vi "Sample in Container.vi"(8 "error in (no error)":errorcluster, 10 "Container":T1, 11 "cRIO-CO2 in":refnum<class "cRIO-CO2.lvclass">) -> (0 "error out":errorcluster, 2 "Sample":refnum<class "Sample.lvclass">, 3 "cRIO-CO2 out":refnum<class "cRIO-CO2.lvclass">)   [LabVIEW 2015, in "cRIO-Carbondioxide.lvlib" / "cRIO-CO2.lvlib" / "cRIO-CO2.lvclass"]
uses:
  cRIO-CO2.lvclass
  Controls/Sample Transfer Container Enumerator.ctl
  subs/Sample/Sample.lvclass
  cRIO-CO2.lvclass/cRIO-CO2.ctl
  Sample Line/Sample Line.lvclass
  Controls/Sample Line State Enumerator.ctl
  CO2 Actor Messages/Ping Msg/Ping Msg.lvclass/Ping Msg.ctl
  <vilib>/ActorFramework/Message Enqueuer/Message Enqueuer.lvclass/Message Enqueuer.ctl
  Storage Line/Storage Line.lvclass
  Storage Line/Storage Line.lvclass/Storage Line.ctl
  Syringe Line/Syringe Line.lvclass
  <vilib>/ActorFramework/Message Enqueuer/Enqueue.vi
  <vilib>/ActorFramework/Message Priority Queue/Priority Enqueue.vi
  <vilib>/ActorFramework/Message Enqueuer/Message Enqueuer.lvclass
  CO2 Actor Messages/Ping Msg/Ping Msg.lvclass
  <vilib>/ActorFramework/Actor/Actor.lvclass
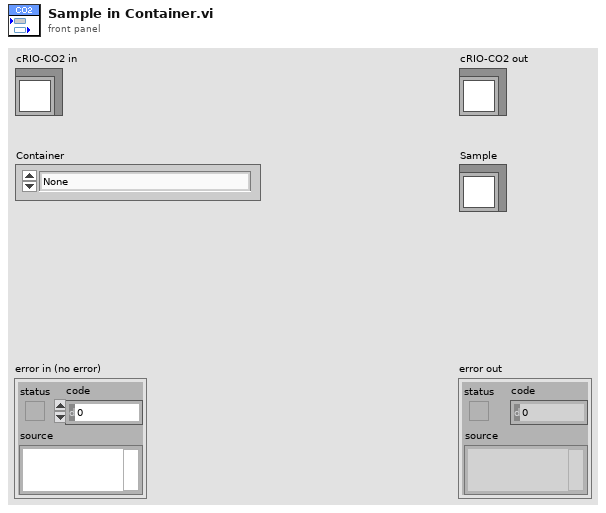
[diagram p1: front panel]
types:
  T1 = typedef "Sample Transfer Container Enumerator.ctl" = enum16{"None", "Sample 1", "Sample 2", "Sample 3", "Sample 4", "Sample 5", "Storage 01", "Storage 02", "Storage 03", "Storage 04", "Storage 05", "Storage 06", "Storage 07", "Storage 08", "Storage 09", "Storage 10", "Storage 11", "Storage 12", "Syringe", "Undefined"}
  T2 = typedef "Sample Line State Enumerator.ctl" = enum16{"All lines closed", "Sample line 1.", "Sample line 2.", "Sample line 3.", "Sample line 4.", "Sample line 5.", "Out of range"}
  T3 = typedef "Dedicated Enqueuers.ctl" = cluster{"Freezers":cluster{"Syringe":refnum<class "Message Enqueuer.lvclass">, "Tank 1":refnum<class "Message Enqueuer.lvclass">, "Tank 2":refnum<class "Message Enqueuer.lvclass">, "Tank 3":refnum<class "Message Enqueuer.lvclass">, "Tank 4":refnum<class "Message Enqueuer.lvclass">}, "Heaters":cluster{"Syringe":refnum<class "Message Enqueuer.lvclass">, "Piston":refnum<class "Message Enqueuer.lvclass">}, "Blowers":cluster{"Tank 1":refnum<class "Message Enqueuer.lvclass">, "Tank 2":refnum<class "Message Enqueuer.lvclass">, "Tank 3":refnum<class "Message Enqueuer.lvclass">, "Tank 4":refnum<class "Message Enqueuer.lvclass">, "Syringe":refnum<class "Message Enqueuer.lvclass">}, "Sample Line":refnum<class "Message Enqueuer.lvclass">, "Storage Line":refnum<class "Message Enqueuer.lvclass">, "Transfer Line":refnum<class "Message Enqueuer.lvclass">, "Syringe Stepper":refnum<class "Message Enqueuer.lvclass">, "Syringe Line":refnum<class "Message Enqueuer.lvclass">, "Capillary Line":refnum<class "Message Enqueuer.lvclass">, "Preparation Line":refnum<class "Message Enqueuer.lvclass">, "Turbo":refnum<class "Message Enqueuer.lvclass">, "Vacuum":refnum<class "Message Enqueuer.lvclass">, "He Line":refnum<class "Message Enqueuer.lvclass">, "Cylinder":refnum<class "Message Enqueuer.lvclass">}
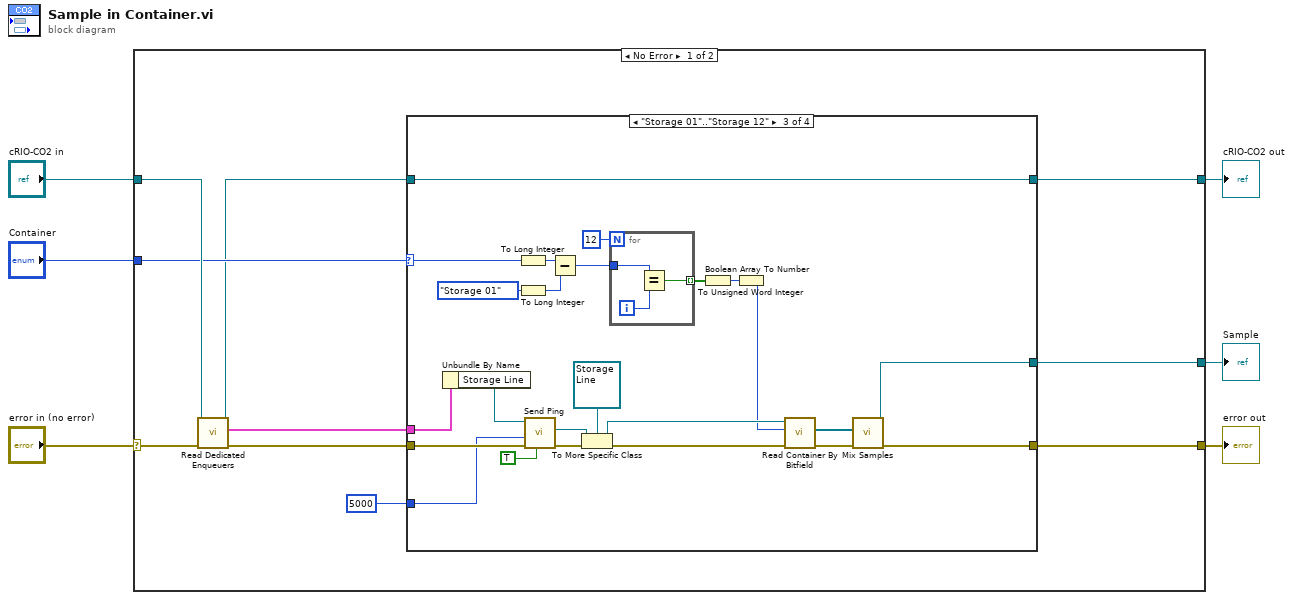
[diagram p0: block diagram]
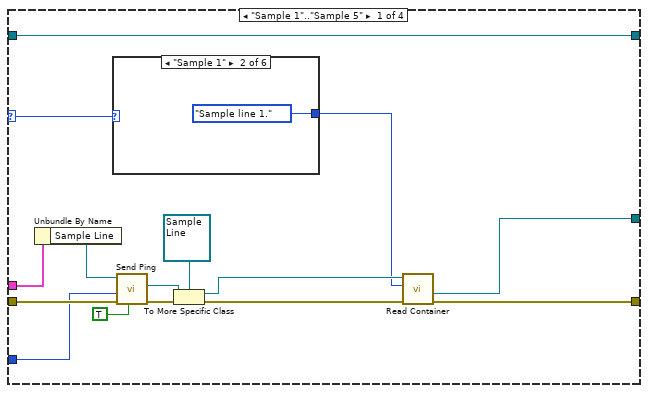
[diagram p2: hidden frame]
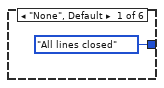
[diagram p3: hidden frame]
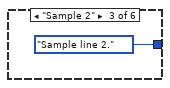
[diagram p4: hidden frame]
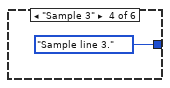
[diagram p5: hidden frame]
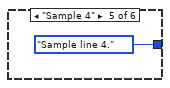
[diagram p6: hidden frame]
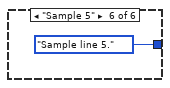
[diagram p7: hidden frame]
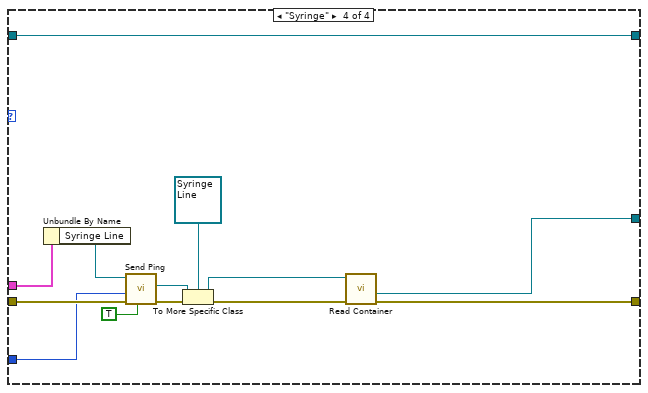
[diagram p9: hidden frame]
diagram:
  n1 = case shown="No Error" "error in (no error)" {
    selector: "error in (no error)" -> [w16 w81]
    tunnel: [w8 w81] -> w5
    tunnel: [w12 w80] -> w3
    tunnel: "cRIO-CO2 in" -> [w15 w80]
    tunnel: "Container" -> [w13 _]
    tunnel: [w7 _] -> w1
    frame No Error {
      n2 = call "Read Dedicated Enqueuers.vi"("error in (no error)"=w16, "cRIO-CO2 in"=w15) -> ("error out"=w14:errorcluster, "Dedicated Enqueuers"=w10:T3, "cRIO-CO2 out"=w11:refnum<class "cRIO-CO2.lvclass">)  [unwired: 6 in, 1 out]
      n3 = case shown="\"Storage 01\"..\"Storage 12\"" w13 {
        selector: w13 -> [w18 _ w49 _]
        tunnel: w14 -> [w30 w39 w59 w76]
        tunnel: [w24 w39 w54 w71] -> w8
        tunnel: [w23 _ w40 w72] -> w7
        tunnel: w10 -> [w31 _ w58 w75]
        tunnel: 5000 ("timeout in ms (1000)") -> [w22 _ w53 w70]
        tunnel: [w21 w38 w52 w69] -> w12
        tunnel: w11 -> [w21 w38 w52 w69]
        frame "Sample 1".."Sample 5" {
          n4 = Unbundle By Name(w31) -> ("Sample Line"=w29:refnum<class "Message Enqueuer.lvclass">)
          n5 = case shown="\"Sample 1\"" w18 {
            tunnel: [Sample_Line_State_Enumerator."All lines closed" ("Sample Line (All Closed)") Sample_Line_State_Enumerator."Sample line 1." ("Sample Line (All Closed)") Sample_Line_State_Enumerator."Sample line 2." ("Sample Line (All Closed)") Sample_Line_State_Enumerator."Sample line 3." ("Sample Line (All Closed)") Sample_Line_State_Enumerator."Sample line 4." ("Sample Line (All Closed)") Sample_Line_State_Enumerator."Sample line 5." ("Sample Line (All Closed)")] -> w17
            frame "None", Default {
            }
            frame "Sample 1" {
            }
            frame "Sample 2" {
            }
            frame "Sample 3" {
            }
            frame "Sample 4" {
            }
            frame "Sample 5" {
            }
          }
          n6 = call "Send Ping.vi"("Return Self (F)"=TRUE, "error in (no error)"=w30, "timeout in ms (1000)"=w22, "Message Enqueuer"=w29) -> ("error out"=w27:errorcluster, "Actor out"=w25:refnum<class "Actor.lvclass">)  [unwired: 4 in, 2 out]
          n7 = To More Specific Class(target class=refnum<class "Sample Line.lvclass"> refnum ("Sample Line in"), reference=w25, error in=w27) -> (specific class reference=w19:refnum<class "Sample Line.lvclass">, error out=w20:errorcluster)
          n8 = call "Read Container.vi"("error in (no error)"=w20, "Sample Line (All Closed)"=w17, "Sample Line in"=w19) -> ("error out"=w24:errorcluster, "Sample"=w23:refnum<class "Sample.lvclass">)  [unwired: 5 in, 2 out]
        }
        frame "None", "Undefined" {
        }
        frame "Storage 01".."Storage 12" {
          n9 = Unbundle By Name(w58) -> ("Storage Line"=w63:refnum<class "Message Enqueuer.lvclass">)
          n10 = To Long Integer(number=w49) -> (32bit integer=w48:i32)
          n11 = To Long Integer(number=Sample_Transfer_Container_Enumerator."Storage 01" ("Container")) -> (32bit integer=w46:i32)
          n12 = call "Send Ping.vi"("Return Self (F)"=TRUE, "error in (no error)"=w59, "timeout in ms (1000)"=w53, "Message Enqueuer"=w63) -> ("error out"=w61:errorcluster, "Actor out"=w60:refnum<class "Actor.lvclass">)  [unwired: 4 in, 2 out]
          n13 = Subtract(x=w48, y=w46) -> (x-y=w45:i32)
          n14 = To More Specific Class(target class=refnum<class "Storage Line.lvclass"> refnum ("Storage Line in"), reference=w60, error in=w61) -> (specific class reference=w51:refnum<class "Storage Line.lvclass">, error out=w50:errorcluster)
          n15 = for {
            N: 12 -> [_]
            tunnel: w45 -> [w65]
            tunnel: [w64] -> w43 mode=indexing
            i -> [w66]
            n16 = Equal?(x=w65, y=w66) -> (x = y?=w64:bool)
          }
          n17 = Boolean Array To Number(Boolean array=w43) -> (number=w42:u32)
          n18 = To Unsigned Word Integer(number=w42) -> (unsigned 16bit integer=w41:u16)
          n19 = call "Read Container By Bitfield.vi"("error in (no error)"=w50, "Bitfield"=w41, "Storage Line in"=w51) -> ("error out"=w56:errorcluster, "Samples"=w55:refnum<class "Sample.lvclass">[])  [unwired: 4 in, 3 out]
          n20 = call "Mix Samples.vi"("error in (no error)"=w56, "Samples In"=w55) -> ("error out"=w54:errorcluster, "Sample out"=w40:refnum<class "Sample.lvclass">)  [unwired: 6 in, 2 out]
        }
        frame "Syringe" {
          n21 = Unbundle By Name(w75) -> ("Syringe Line"=w79:refnum<class "Message Enqueuer.lvclass">)
          n22 = call "Send Ping.vi"("Return Self (F)"=TRUE, "error in (no error)"=w76, "timeout in ms (1000)"=w70, "Message Enqueuer"=w79) -> ("error out"=w78:errorcluster, "Actor out"=w77:refnum<class "Actor.lvclass">)  [unwired: 4 in, 2 out]
          n23 = To More Specific Class(target class=refnum<class "Syringe Line.lvclass"> refnum ("Syringe Line in"), reference=w77, error in=w78) -> (specific class reference=w68:refnum<class "Syringe Line.lvclass">, error out=w67:errorcluster)
          n24 = call "Read Container.vi"("error in (no error)"=w67, "Syringe Line in"=w68) -> ("error out"=w71:errorcluster, "Sample"=w72:refnum<class "Sample.lvclass">)  [unwired: 6 in, 2 out]
        }
      }
    }
    frame Error {
    }
  }
  "error out" <- w5
  "cRIO-CO2 out" <- w3
  "Sample" <- w1
